vi "fgv_Z_parameters.vi"(8 "error in (no error)":errorcluster, 10 "Function":enum16{"Intialize", "Write", "Read", "Clear"}(ring), 11 "Z Parameters":T1) -> (0 "error out":errorcluster, 3 "Z Parameters":T1)   [LabVIEW 2020]
panel:
  # "SUBROUTINE"
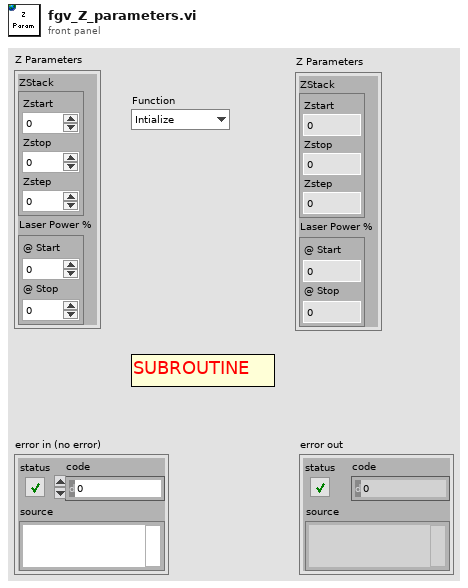
[diagram p1: front panel]
types:
  T1 = cluster{"ZStack":cluster{"Zstart":dbl, "Zstop":dbl, "Zstep":dbl}, "Laser Power %":cluster{"@ Start":dbl, "@ Stop":dbl}}
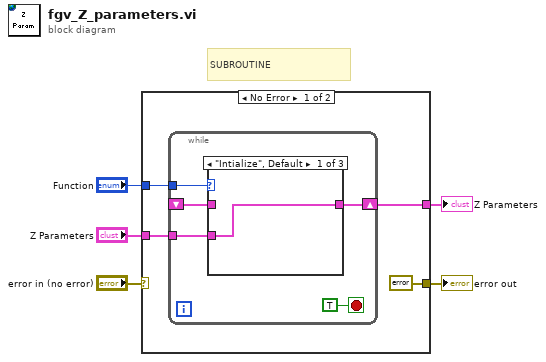
[diagram p0: block diagram]
diagram:
  # "SUBROUTINE"
  n1 = case shown="No Error" "error in (no error)" {
    selector: "error in (no error)" -> [_ w18]
    tunnel: "Function" -> [w9 _]
    tunnel: [w8 w19] -> w3
    tunnel: "Z Parameters" -> [w7 w19]
    tunnel: [errorcluster {"status"=FALSE, "code"=0, "source"=""} ("error IO") w18] -> w1
    frame No Error {
      n2 = while {
        tunnel: w9 -> [w13]
        tunnel: w7 -> [w11]
        shift-right: [w12] -> w8
        shift-left: _ -> [w10]
        stop <- TRUE stop-if-true
        n3 = case shown="\"Intialize\", Default" w13 {
          tunnel: [w15 w16 w17] -> w12
          tunnel: w11 -> [w15 w16 _]
          tunnel: w10 -> [_ _ w17]
          frame "Intialize", Default {
          }
          frame "Write" {
          }
          frame "Read" {
          }
        }
      }
    }
    frame Error {
    }
  }
  "error out" <- w1
  "Z Parameters" <- w3
